vi "MagnaDC Read Volts Amps.vi"(8 "error in (no error)":errorcluster, 11 "VISA resource name":refnum<visa-resource-name>="TCPIP0::131.227.181.163::50505::SOCKET") -> (0 "error out":errorcluster, 2 "Current (A)":dbl=0.2, 3 "Voltage (V)":dbl=203.0)   [LabVIEW 2022 SP3]
doc: "Simple example how to control power supplu output using voltage and current levels."
uses:
  Magna sub vis/MagnaDC.lvlib
panel:
  # "(c) 2004 - 2018 Magna-Power Electronics Inc.  ALL RIGHTS RESERVED."
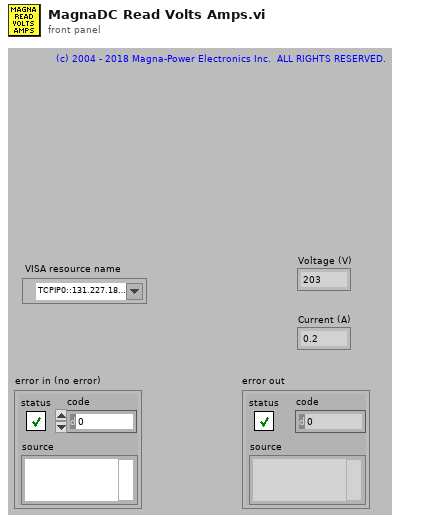
[diagram p1: front panel]
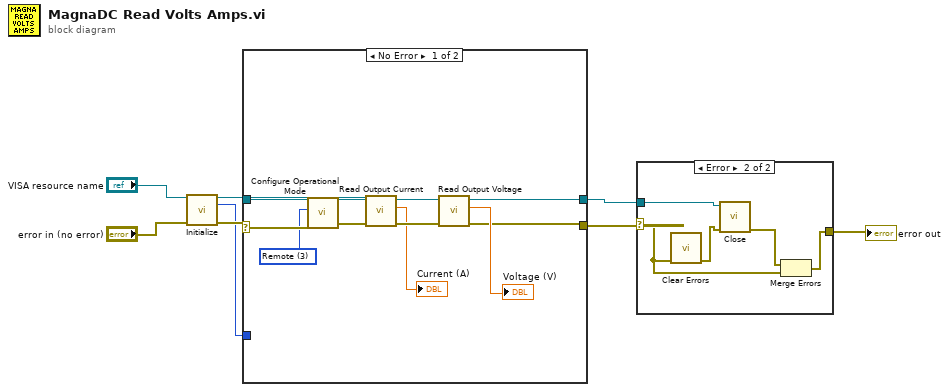
[diagram p0: block diagram]
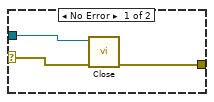
[diagram p2: hidden frame]
diagram:
  n1 = call "Initialize.vi"("VISA resource name"="VISA resource name", "error in (no error)"="error in (no error)") -> ("VISA resource name out"=w6:refnum<visa-resource-name>, "Modulation Available"=w3:u32, "error out"=w7:errorcluster)  [unwired: 10 in, 1 out]
  n2 = case shown="No Error" w7 {
    selector: w7 -> [w18 w21]
    tunnel: w6 -> [w19 w20]
    tunnel: [w12 w21] -> w5
    tunnel: [w11 w20] -> w4
    tunnel: w3 -> [_ _]
    frame No Error {
      w17 = u32 3 items=["Rotary", "Keypad", "Ext Pgm", "Remote"] ("Operational Mode")
      n3 = call "Configure Operational Mode.vi"("error in (no error)"=w18, "Operational Mode"=w17, "VISA resource name"=w19) -> ("error out"=w9:errorcluster, "VISA resource name out"=w10:refnum<visa-resource-name>)  [unwired: 7 in]
      n4 = call "Read Output Current.vi"("error in (no error)"=w9, "VISA resource name"=w10) -> ("error out"=w15:errorcluster, "Actual Current Level (A)"=→"Current (A)":dbl, "VISA resource name out"=w14:refnum<visa-resource-name>)  [unwired: 6 in]
      n5 = call "Read Output Voltage.vi"("error in (no error)"=w15, "VISA resource name"=w14) -> ("error out"=w12:errorcluster, "Actual Voltage Level (V)"=→"Voltage (V)":dbl, "VISA resource name out"=w11:refnum<visa-resource-name>)  [unwired: 7 in]
    }
    frame Error {
    }
  }
  n6 = case shown="Error" w5 {
    selector: w5 -> [w24 w26]
    tunnel: [w22 w25] -> w1
    tunnel: w4 -> [w23 w28]
    frame No Error {
      n7 = call "Close.vi"("error in (no error)"=w24, "VISA resource name"=w23) -> ("error out"=w22:errorcluster)  [unwired: 9 in]
    }
    frame Error {
      n8 = call <vilib>:"Clear Errors.vi"("error in (no error)"=w26) -> ("error out"=w29:errorcluster)  [unwired: 5 in, 1 out]
      n9 = call "Close.vi"("error in (no error)"=w29, "VISA resource name"=w28) -> ("error out"=w27:errorcluster)  [unwired: 9 in]
      n10 = Merge Errors(w27, w26) -> (w25:errorcluster)
    }
  }
  "error out" <- w1
